vi "CHECK_HOT.vi"(10 "argv":string[](array[string]), 11 "args":u8) -> ()   [LabVIEW 2014]
uses:
  TORC Code/GlobalVariable.vi
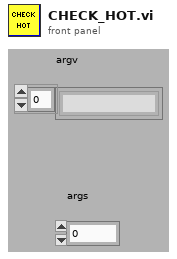
[diagram p1: front panel]
types:
  T1 = typedef "WPI_DigitalInputDevRef.ctl" = cluster{"DevStatus":errorcluster, "DIO Channel":T2, "Controller":T3}
  T2 = typedef "FPGA_DIOChannel.ctl" = enum8{"DIO 0", "DIO 1", "DIO 2", "DIO 3", "DIO 4", "DIO 5", "DIO 6", "DIO 7", "DIO 8", "DIO 9", "DIO MXP 0", "DIO MXP 1", "DIO MXP 2", "DIO MXP 3", "DIO MXP 4", "DIO MXP 5", "DIO MXP 6", "DIO MXP 7", "DIO MXP 8", "DIO MXP 9", "DIO MXP 10", "DIO MXP 11", "DIO MXP 12", "DIO MXP 13", "DIO MXP 14", "DIO MXP 15", "Invalid"}
  T3 = typedef "FPGA_TypedefDigitalModule.ctl" = enum16{"Controller 1"}
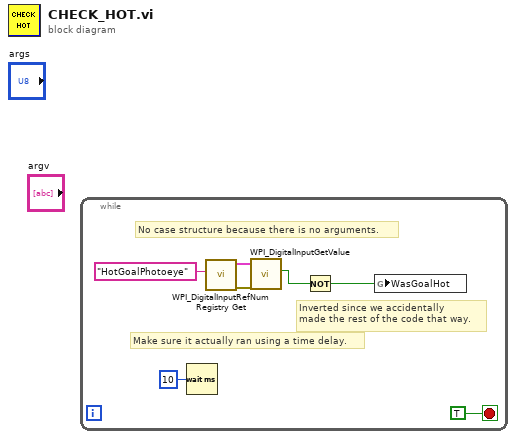
[diagram p0: block diagram]
diagram:
  n1 = while {
    stop <- TRUE stop-if-true
    # "Inverted since we accidentally\nmade the rest of the code that way."
    # "No case structure because there is no arguments."
    # "Make sure it actually ran using a time delay."
    n2 = Wait (ms)(milliseconds to wait=u32 10) -> ()  [unwired: 1 out]
    n3 = call <vilib>:"WPI_DigitalInputRefNum Registry Get.vi"("refnum name"="HotGoalPhotoeye") -> ("error out"=w6:errorcluster, "DigitalInputDevRef"=w5:T1)  [unwired: 9 in]
    n4 = call <vilib>:"WPI_DigitalInputGetValue.vi"("error in (no error)"=w6, "DigitalInputDevRef"=w5) -> ("Value"=w4:bool)  [unwired: 7 in, 2 out]
    n5 = Not(x=w4) -> (.not. x?=w1:bool)
    n6 = global write "GlobalVariable.vi" "WasGoalHot"(w1) -> ()
  }
